vi "Constants.vi"() -> ()   [LabVIEW 2020, in "AIM ARINC 429 Scripting.lvlib"]
doc: "Use this Global VI to access the GUIDs assigned to the page resources of the Custom Device."
uses:
  AIM ARINC 429 Scripting.lvlib
panel:
  in  "Tab Control":enum32{"GUIDs", "Constants", "Properties"}(tab)
  in  "GUID.Logging":string="A7E97344-F434-4F0B-98D8-9CD4B5E268FA"
  in  "GUID.Status Channel":string="F1643FA0-1C8B-4412-B885-8686A95466A9"
  in  "GUID.Status":string="8E884AA6-4EB7-4451-9366-671B1F80E122"
  in  "GUID.Channel Specification":string="B2A2CF05-6E12-4B12-AD6E-484715D7E6DB"
  in  "GUID.Receive Time":string="8384C54A-C815-4431-A5F1-A0B3A5E0000E"
  in  "GUID.Word":string="F4424C32-A6E9-4D92-92EF-32D1787FC962"
  in  "GUID.Parameter":string="C134BE96-2099-43AB-94FA-9B4420FA681F"
  in  "GUID.Import Frames":string="0697C98A-9CCE-47AB-B6F9-386AC77E8880"
  in  "GUID.Outgoing":string="4820ED19-BA5E-4F93-B9FD-0537F273FAE4"
  in  "GUID.Incoming":string="D51C55E8-15D6-4FA2-852D-BCEC3384A3F2"
  in  "GUID.Database":string="0E05AB3D-2EA9-4234-944A-B8CBACBD7759"
  in  "GUID.Add Database":string="D7790871-F68E-4527-B8AD-D6388CFBE356"
  in  "GUID.Port":string="8F4E2FDB-ABCC-4261-A817-85981E70FAF8"
  in  "GUID.Add Port":string="4DC2F88C-216B-4D3D-990A-E6D477C716D8"
  in  "GUID.Configuration Files":string="9CC1718D-5483-4E02-9349-BDEBD161B45E"
  in  "GUID.Ports":string="758B4561-0065-41D8-A3C5-EE4D6DBA4B41"
  in  "GUID.Protocol":string="DE6C4FDC-BD63-4F5C-9E61-946DAF30A276"
  in  "GUID.Vendor":string="55C1F7F6-C65E-44A3-892F-ED507C2CC731"
  in  "GUID.Label":string="ADB9C5E2-6464-4FCC-92F3-599E637ADE1E"
  in  "GUID.AIM ARINC 429":string="2D790D37-75CB-4384-9C8B-614C6F0F16DF"
  in  "Logging":string="Logging"
  in  "Timestamp":string="Timestamp"
  in  "Parameters Cfg File":string="error_key_parameters_config_file"
  in  "Hardware Cfg File":string="error_key_hardware_config_file"
  in  "Parameters Cfg MD5":string="error_key_parameters_config_MD5"
  in  "Trigger":string="Trigger"
  in  "Disable":string="Disable"
  in  "Status":string="Status"
  in  "PXI Slot Number":string="PXI Slot Number"
  in  "Card Number":string="Card Number"
  in  "Channel":string="Channel"
  in  "Import Frames":string="Import Frames"
  in  "Frame":string="Frame"
  in  "Outgoing":string="Outgoing"
  in  "Incoming":string="Incoming"
  in  "Add Database":string="Add Database"
  in  "Database":string="Database"
  in  "Port":string="Port"
  in  "Add Port":string="Add Port"
  in  "Configuration Files":string="Configuration Files"
  in  "Ports":string="Ports"
  in  "Prop.Logging.File Name Timestamp":string="File Name Timestamp"
  in  "Prop.Logging.File":string="File"
  in  "Prop.Logging.Data Word Format":string="Data Word Format"
  in  "Prop.Logging.Enabled":string="Enabled"
  in  "Prop.Logging.Directory":string="Log Directory"
  in  "Prop.MD5.Checksum":string="MD5.Checksum"
  in  "Prop.Timeout.Error.Count":string="Timeout Error Count"
  in  "Prop.Bit.Timing.Error.Count":string="Bit Timing Error Count"
  in  "Prop.Long.Word.Error.Count":string="Long Word Error Count"
  in  "Prop.Parity.Error.Count":string="Parity Error Count"
  in  "Prop.Gap.Error.Count":string="Gap Error Count"
  in  "Prop.Receiving.Error.Count":string="Receiving Error Count"
  in  "Prop.Hardware.Configuration.File":string="Hardware Configuration File"
  in  "Prop.Parameters.Needed":string="Parameters File Needed"
  in  "Prop.Parameters.File":string="Win Parameters File Path"
  in  "Prop.Hardware.File":string="Win File Path"
  in  "Prop.PXI.Slot.Number":string="PXI Slot Number"
  in  "Prop.Initialization.Method":string="Initialization Method"
  in  "Prop.Core.Number":string="core number"
  in  "Prop.Card.Number":string="card number"
  in  "Prop.Asynchronous.Loop.Time":string="Asynchronous Loop Time"
  in  "Prop.xml.Name":string="xmlName"
  in  "Prop.Database.Path":string="Database.Path"
  in  "Prop.Database.Name":string="Database.Name"
  in  "Prop.Frame.ID":string="Frame.ID"
  in  "Prop.Compiled.Settings":string="Compiled.Settings"
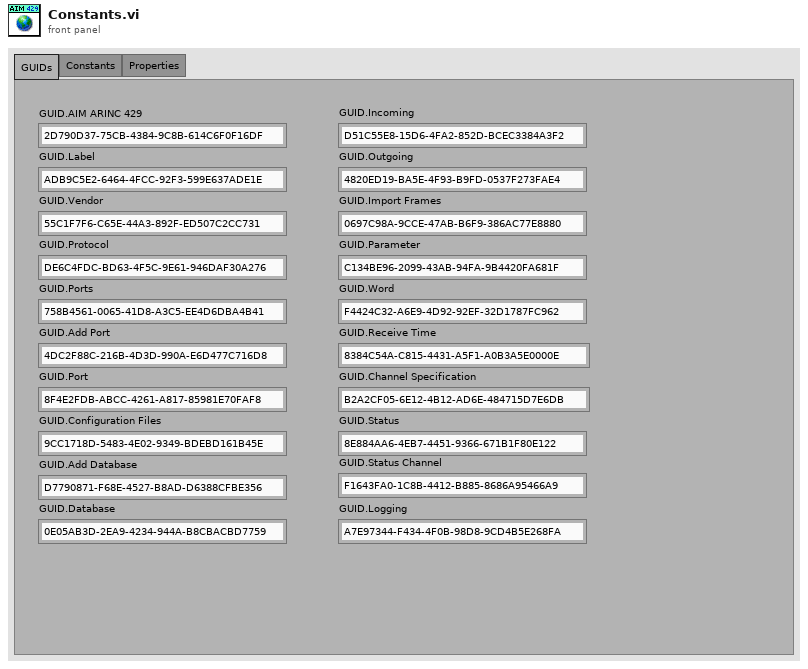
[diagram p1: front panel]
diagram:
